vi "PIParams.vi"(10 "PI parameters":T1) -> (2 "Params Out":string[](array[string]))   [LabVIEW 2018]
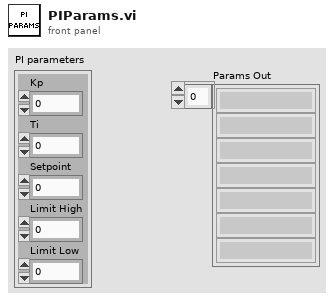
[diagram p1: front panel]
types:
  T1 = cluster{"Kp":dbl, "Ti":dbl, "Setpoint":dbl, "Limit High":dbl, "Limit Low":dbl}
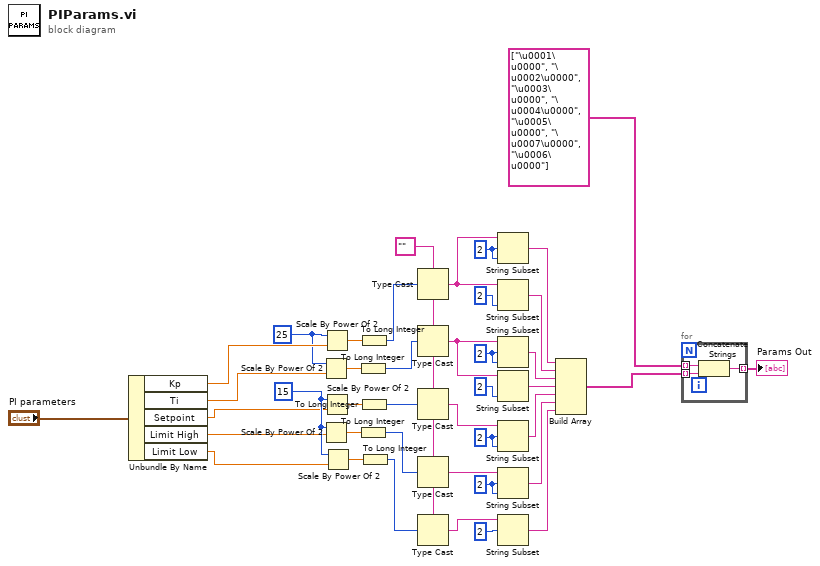
[diagram p0: block diagram]
diagram:
  w4 = "" ("data in")
  w23 = 2 ("length (rest)")
  w24 = 2 ("length (rest)")
  w15 = 2 ("length (rest)")
  w14 = 2 ("length (rest)")
  w33 = 15
  w36 = 25
  n1 = Unbundle By Name("PI parameters") -> ("Kp"=w39:dbl, "Ti"=w37:dbl, "Setpoint"=w32:dbl, "Limit High"=w31:dbl, "Limit Low"=w30:dbl)
  n2 = Scale By Power Of 2(n=w36, x=w37) -> (x*2^n=w38:dbl)
  n3 = Scale By Power Of 2(n=w33, x=w31) -> (x*2^n=w35:dbl)
  n4 = Scale By Power Of 2(n=w36, x=w39) -> (x*2^n=w41:dbl)
  n5 = Scale By Power Of 2(n=w33, x=w32) -> (x*2^n=w34:dbl)
  n6 = Scale By Power Of 2(n=w33, x=w30) -> (x*2^n=w29:dbl)
  n7 = To Long Integer(number=w38) -> (32bit integer=w8:i32)
  n8 = To Long Integer(number=w35) -> (32bit integer=w6:i32)
  n9 = To Long Integer(number=w41) -> (32bit integer=w9:i32)
  n10 = To Long Integer(number=w34) -> (32bit integer=w7:i32)
  n11 = To Long Integer(number=w29) -> (32bit integer=w5:i32)
  n12 = Type Cast(type=w4, x=w9) -> (*(type *) &x=w10:string)
  n13 = Type Cast(type=w4, x=w8) -> (*(type *) &x=w13:string)
  n14 = Type Cast(type=w4, x=w7) -> (*(type *) &x=w21:string)
  n15 = Type Cast(type=w4, x=w6) -> (*(type *) &x=w17:string)
  n16 = Type Cast(type=w4, x=w5) -> (*(type *) &x=w18:string)
  n17 = String Subset(string=w10, offset (0)=w14, length (rest)=w14) -> (substring=w27:string)
  n18 = String Subset(string=w10, length (rest)=2 ("length (rest)")) -> (substring=w28:string)  [unwired: 1 in]
  n19 = String Subset(string=w13, offset (0)=w15, length (rest)=w15) -> (substring=w26:string)
  n20 = String Subset(string=w13, length (rest)=2 ("length (rest)")) -> (substring=w25:string)  [unwired: 1 in]
  n21 = String Subset(string=w21, offset (0)=w24, length (rest)=w24) -> (substring=w16:string)
  n22 = String Subset(string=w17, offset (0)=w23, length (rest)=w23) -> (substring=w20:string)
  n23 = String Subset(string=w18, offset (0)=2 ("length (rest)")) -> (substring=w19:string)  [unwired: 1 in]
  n24 = Build Array(w27, w28, w26, w25, w16, w20, w19) -> (w2:string[])
  n25 = for {
    tunnel: string[] ["\u0001\u0000", "\u0002\u0000", "\u0003\u0000", "\u0004\u0000", "\u0005\u0000", "\u0007\u0000", "\u0006\u0000"] ("data in") -> [w44] mode=indexing
    tunnel: w2 -> [w43] mode=indexing
    tunnel: [w42] -> w1 mode=indexing
    n26 = Concatenate Strings(w44, w43) -> (w42:string)
  }
  "Params Out" <- w1
